vi "Main-PSD+EQP_YCC.vi"() -> ()   [LabVIEW 2014]
uses:
  Main-Stage-PI/(Global) Current handle and LaserPower_YCC.vi
  <vilib>/DAQmx/create/channels.llb/DAQmx Create Channel (AI-Voltage-Basic).vi
  <vilib>/DAQmx/configure/timing.llb/DAQmx Timing (Sample Clock).vi
  <vilib>/DAQmx/read.llb/DAQmx Read (Analog 2D DBL NChan NSamp).vi
panel:
  in  "Notch Filter On?":bool
  out "QPD raw(V) xyz":dbl[][](array[numeric])
  out "kx (pN/nm)":dbl
  in  "Who's Data":enum16{"YCC", "PYW", "LCH", "YYH"}(ring)
  in  "Save?":bool
  out "Frequency (Hz)\n0,df, 2df,...(n/2-1)Fs":dbl[](array[numeric])
  in  "Temperature (C)":dbl=22.0
  out "df (freq. resolution) Hz":dbl
  in  "record time per cycle (s)":dbl=0.125
  in  "EQP on?":bool
  out "Beta (V/um)":dbl[](array[numeric])
  out "Varicance (V^2)":dbl[](array[numeric])
  out "y-variance (V)":dbl format="%0.2f"
  out "x-variance (V)":dbl format="%0.2f"
  out "Y-conversion factor (V/um)":dbl
  out "X-conversion factor (V/um)":dbl
  out "EQP-Trap Stiffness (pN/nm)":dbl[](array[numeric])
  out "best fit parameters-y":dbl[](array[numeric])
  out "best fit parameters-z":dbl[](array[numeric])
  out "best fit parameters-x":dbl[](array[numeric])
  in  "Fit z?":bool
  in  "Fit y?":bool
  out "best nonlinear fit PSDz":dbl[](array[numeric])
  out "best nonlinear fit PSDy":dbl[](array[numeric])
  out "best nonlinear fit PSDx":dbl[](array[numeric])
  in  "Custum Fs (Hz)":i32
  in  "Focal shift factor":dbl=1.22
  out "best fit parameters":dbl[][](array[numeric])
  out "kx/kz":dbl
  in  "Freq End Cut":dbl=60000.0
  in  "Freq Strat Cut":dbl=10.0
  out "Trap Stiffness (pN/nm)":dbl[](array[numeric])
  in  "bead height (um)":dbl=2.0
  in  "bead radius (um)":dbl=0.515
  out "PSDz":dbl[](array[numeric])
  out "PSDy":dbl[](array[numeric])
  out "PSDx":dbl[](array[numeric])
  out "Frequency (Hz)\n0,df, 2df,...1/2Fs":dbl[](array[numeric])
  in  "Tab Control":enum32{"PSD x & y", "PSD x & z"}(tab)
  out "PSD x & y":T1(graph)
  out "PSD x & z":T2(graph)
  out "Corner Frequency (Hz)\n(fx,fy,fz)":dbl[](array[numeric])
  in  "Fit Lorentz PSD?":bool=TRUE
  out "Avg. PSD":dbl[][](array[numeric])
  out "# of PSD sum":i32
  in  "# of PSD Avg.":dbl=50.0
  in  "stop to fit":bool
  in  "T=NI made PSD\nF=YCC made PSD":bool
  out "Sampling rate (Hz)":i32
  in  "physical channels":tag="Dev2/ai2, Dev2/ai0, Dev2/ai16"
  in  "Sampling Rate (Hz)":T3(ring)=enum."131072"
  # "Fc=80k for fs=131072Hz"
  # "x"
  # "y"
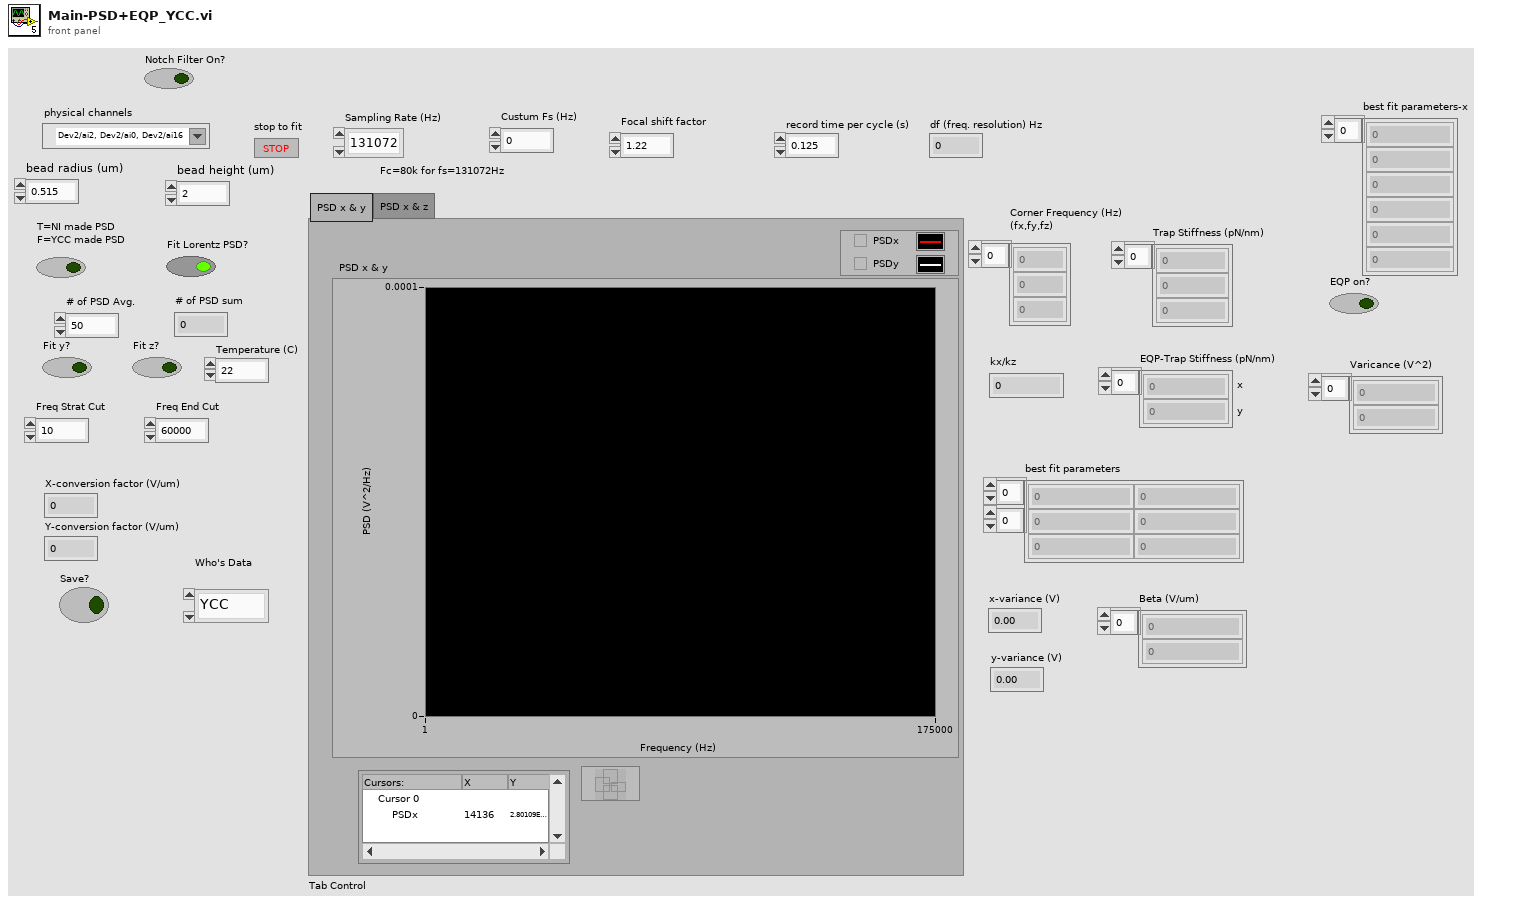
[diagram p1: front panel]
types:
  T1 = cluster{"Frequency (Hz)\ndf, 2df,...1/2Fs":dbl[], "PSDy":dbl[]}[]
  T2 = cluster{"Frequency (Hz)\ndf, 2df,...1/2Fs":dbl[], "PSDz":dbl[]}[]
  T3 = enum16{"custum", "16384", "32768", "65536", "131072", "262144"}
  T4 = cluster{"Frequency (Hz)\n0,df, 2df,...1/2Fs":dbl[], "PSDx":dbl[]}
  T5 = cluster{"Frequency (Hz)\n0,df, 2df,...1/2Fs":dbl[], "PSDz":dbl[]}
  T6 = cluster{"Frequency (Hz)\n0,df, 2df,...1/2Fs":dbl[], "PSDy":dbl[]}
  T7 = cluster{"Frequency (Hz)\n0,df, 2df,...1/2Fs":dbl[], "PSDz":dbl[]}[]
  T8 = cluster{"Frequency (Hz)\n0,df, 2df,...1/2Fs":dbl[], "PSDy":dbl[]}[]
  T9 = cluster{"Frequency (Hz)\n0,df, 2df,...1/2Fs":dbl[], "best nonlinear fit PSDz":dbl[]}
  T10 = cluster{"Frequency (Hz)\n0,df, 2df,...1/2Fs":dbl[], "best nonlinear fit PSDx":dbl[]}
  T11 = cluster{"Frequency (Hz)\n0,df, 2df,...1/2Fs":dbl[], "best nonlinear fit PSDy":dbl[]}
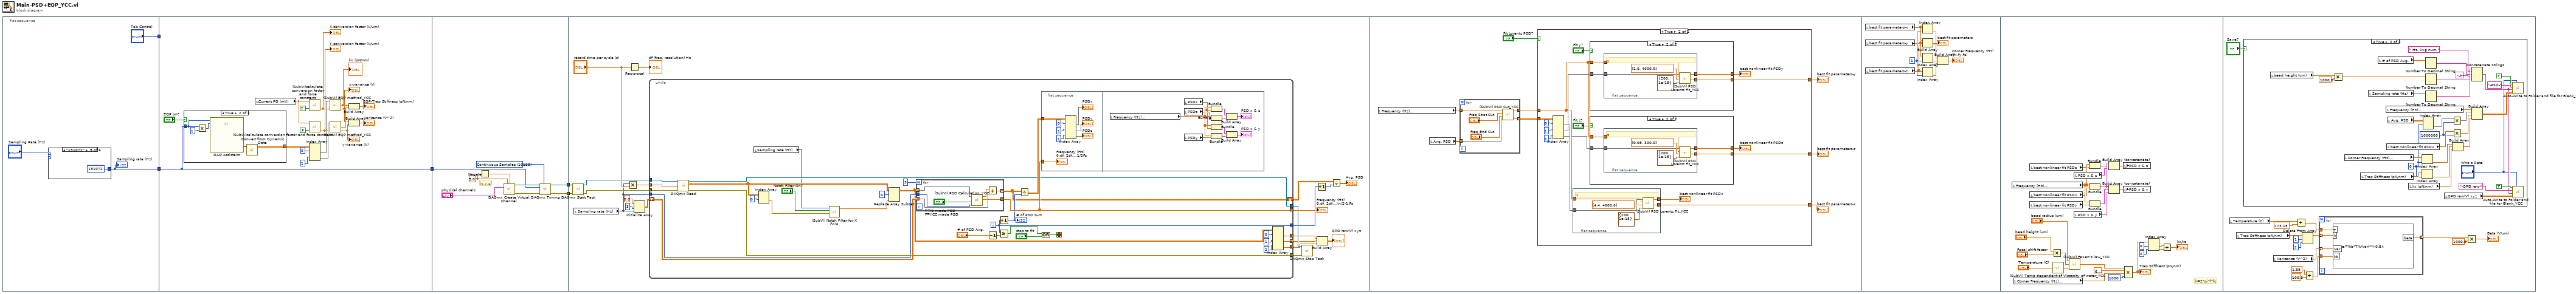
[diagram p0: block diagram]
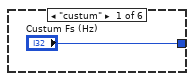
[diagram p2: hidden frame]
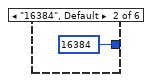
[diagram p3: hidden frame]
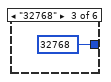
[diagram p4: hidden frame]
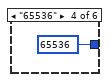
[diagram p5: hidden frame]
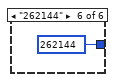
[diagram p6: hidden frame]
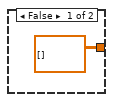
[diagram p7: hidden frame]
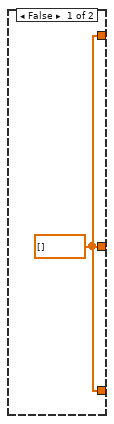
[diagram p8: hidden frame]
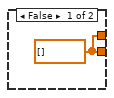
[diagram p9: hidden frame]
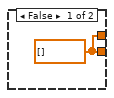
[diagram p10: hidden frame]
diagram:
  n1 = flat-sequence {
    tunnel: [w7] -> w3
    tunnel: ["Tab Control"] -> w1
    tunnel: w3 -> [w32]
    tunnel: [w32] -> w2
    tunnel: w1 -> [_]
    tunnel: w2 -> [w45]
    tunnel: [w42] -> w5
    tunnel: [w41] -> w4
    tunnel: w5 -> [w69]
    tunnel: w4 -> [w68]
    frame #0 {
      n2 = case shown="\"131072\"" "Sampling Rate (Hz)" {
        tunnel: ["Custum Fs (Hz)" 16384 32768 65536 131072 262144] -> w7
        frame "custum" {
        }
        frame "16384", Default {
        }
        frame "32768" {
        }
        frame "65536" {
        }
        frame "131072" {
        }
        frame "262144" {
        }
      }
      "Sampling rate (Hz)" <- w7
    }
    frame #1 {
      n3 = case shown="True" "EQP on?" {
        tunnel: w32 -> [_ w38]
        tunnel: [dbl[][] [] ("Array") w34] -> w21
        frame False {
        }
        frame True {
          n4 = Multiply(x=w38, y=1) -> (x*y=w36:i32)
          n5 = call "DAQ Assistant"("rate"=w38, "number of samples"=w36) -> ("data"=w35:dynamicdata)  [unwired: 15 in, 2 out]
          n6 = call "Convert from Dynamic Data"("Dynamic Data Type"=w35) -> ("Array"=w34:dbl[][])  [unwired: 3 in]
        }
      }
      n7 = global read "(Global) Current handle and LaserPower_YCC.vi" "Current PD (mV)"() -> (w18:dbl)
      n8 = Index Array(array=w21, index (row) #1=0 ("index (row)"), index (row) #2=1 ("index (row)")) -> (element #1=w29:dbl[], element #2=w28:dbl[])  [unwired: 2 in]
      n9 = call "(SubVI)calculate conversion factor and force constant.vi"("X=T\nY=F"=TRUE ("X=T\nY=F"), "laser power (mW)"=w18) -> ("conversion factor (V/um)"=w17:dbl)  [unwired: 2 in, 1 out]
      "X-conversion factor (V/um)" <- w17
      n10 = call "(SubVI)calculate conversion factor and force constant.vi"("X=T\nY=F"=FALSE ("X=T\nY=F"), "laser power (mW)"=w18) -> ("conversion factor (V/um)"=w19:dbl)  [unwired: 2 in, 1 out]
      "Y-conversion factor (V/um)" <- w19
      n11 = call "(SubVI) EQP method_YCC.vi"("Sensitivity (V/um)"=w17, "position (V)"=w29) -> ("variance (V)"=w24:dbl, "k (pN/nm)"=w27:dbl)  [unwired: 2 in]
      "x-variance (V)" <- w24
      "kx (pN/nm)" <- w27
      n12 = call "(SubVI) EQP method_YCC.vi"("Sensitivity (V/um)"=w19, "position (V)"=w28) -> ("variance (V)"=w23:dbl, "k (pN/nm)"=w26:dbl)  [unwired: 2 in]
      "y-variance (V)" <- w23
      n13 = Build Array(w27, w26) -> (→"EQP-Trap Stiffness (pN/nm)":dbl[])
      n14 = Build Array(w24, w23) -> (→"Varicance (V^2)":dbl[])
    }
    frame #2 {
      w40 = 5.0 ("maximum value")
      w43 = 10123 items=["Finite Samples"=10178, "Continuous Samples"=10123, "Hardware Timed Single Point"=12522] ("sample mode")
      # "(x,y,z)"
      n15 = Negate(x=w40) -> (-x=w39:dbl)
      n16 = call-poly <vilib>:"DAQmx Create Virtual Channel.vi"("maximum value"=w40, "minimum value"=w39, "physical channels"="physical channels") -> ("task out"=w46:refnum<k21>, "error out"=w44:errorcluster)  [unwired: 11 in]
      n17 = call-poly <vilib>:"DAQmx Timing.vi"("task/channels in"=w46, "sample mode"=w43, "rate"=w45, "error in"=w44) -> ("task out"=w42:refnum<k21>, "error out"=w41:errorcluster)  [unwired: 10 in]
    }
    frame #3 {
      n18 = call <vilib>:"DAQmx Start Task.vi"("task/channels in"=w69, "error in"=w68) -> ("task out"=w67:refnum<k21>, "error out"=w66:errorcluster)  [unwired: 12 in]
      n19 = local read "Sampling rate (Hz)"() -> (w52:i32)
      n20 = Multiply(x=w52, y="record time per cycle (s)") -> (x*y=w55:dbl)
      n21 = Reciprocal(x="record time per cycle (s)") -> (1/x=→"df (freq. resolution) Hz":dbl)
      n22 = Initialize Array(0.0 ("element"), 3 ("dimension size"), w52) -> (w63:dbl[][])
      n23 = while {
        tunnel: w67 -> [w101]
        tunnel: w66 -> [w100]
        shift-right: [w86] -> w56
        shift-left: w63 -> [w99]
        tunnel: [w90] -> w59
        tunnel: w55 -> [w85]
        tunnel: [w91] -> w62
        tunnel: [w89] -> w58
        tunnel: [w88] -> w57
        tunnel: w52 -> [w84]
        tunnel: [w80] -> w51 mode=concatenating
        tunnel: [w79] -> w50 mode=concatenating
        tunnel: [w78] -> w49 mode=concatenating
        i -> [w91]
        stop <- w94 stop-if-true
        n24 = call-poly <vilib>:"DAQmx Read.vi"("task/channels in"=w101, "number of samples per channel"=w85, "error in"=w100) -> ("task out"=w89:refnum<k21>, "data"=w75:dbl[][], "error out"=w88:errorcluster)  [unwired: 10 in]
        n25 = local read "Sampling rate (Hz)"() -> (w72:i32)
        n26 = Index Array(array=w75, index (row)=0) -> (element=w70:dbl[])  [unwired: 1 in]
        n27 = call "(SubVI) Notch Filter for X Axis.vi"("Sampling rate (Hz)"=w72, "Notch Filter On?"="Notch Filter On?", "data"=w70) -> ("Filtered Data"=w73:dbl[])  [unwired: 5 in]
        n28 = Replace Array Subset(array=w75, new element=w73, index (row)=0) -> (w74:dbl[][])  [unwired: 1 in]
        n29 = for {
          N: 3 -> [_]
          tunnel: w74 -> [w126] mode=indexing
          tunnel: w84 -> [w120]
          tunnel: [w123] -> w90
          tunnel: [w122] -> w86 mode=indexing
          tunnel: w99 -> [w121] mode=indexing
          n30 = call "(SubVI) PSD Calculation_YCC.vi"("sampling frequency (Hz)"=w120, "T=NI made PSD\nF=YCC made PSD"="T=NI made PSD\nF=YCC made PSD", "QPD data"=w126) -> ("Frequency (Hz)\n0,df, 2df,...(n/2-1)Fs"=w123:dbl[], "Power Spectrum (V^2 rms) (V^2/Hz)"=w124:dbl[])  [unwired: 3 in]
          n31 = Add(x=w124, y=w121) -> (x+y=w122:dbl[])
        }
        n32 = Decrement(x="# of PSD Avg.") -> (x-1=w96:dbl)
        n33 = Increment(x=w91) -> (x+1=w87:i32)
        "# of PSD sum" <- w87
        n34 = Greater Or Equal?(x=w91, y=w96) -> (x >= y?=w95:bool)
        n35 = Divide(x=w86, y=w87) -> (x/y=w92:dbl[][])
        n36 = Or(x=w95, y="stop to fit") -> (x .or. y?=w94:bool)
        n37 = flat-sequence {
          tunnel: w92 -> [w106]
          tunnel: w90 -> [w103]
          frame #0 {
            n38 = Index Array(array=w106, index (row) #1=0 ("index (row)"), index (row) #2=1 ("index (row)"), index (row) #3=2 ("index (row)")) -> (element #1=→"PSDx":dbl[], element #2=→"PSDy":dbl[], element #3=→"PSDz":dbl[])  [unwired: 3 in]
            "Frequency (Hz)\n0,df, 2df,...1/2Fs" <- w103
          }
          frame #1 {
            n39 = local read "Frequency (Hz)\n0,df, 2df,...1/2Fs"() -> (w115:dbl[])
            n40 = local read "PSDx"() -> (w110:dbl[])
            n41 = local read "PSDz"() -> (w111:dbl[])
            n42 = local read "PSDy"() -> (w116:dbl[])
            n43 = Bundle("Frequency (Hz)\n0,df, 2df,...1/2Fs"=w115, "PSDx"=w110) -> (w113:T4)  [unwired: 1 in]
            n44 = Bundle("Frequency (Hz)\n0,df, 2df,...1/2Fs"=w115, "PSDz"=w111) -> (w112:T5)  [unwired: 1 in]
            n45 = Bundle("Frequency (Hz)\n0,df, 2df,...1/2Fs"=w115, "PSDx"=w110) -> (w117:T4)  [unwired: 1 in]
            n46 = Bundle("Frequency (Hz)\n0,df, 2df,...1/2Fs"=w115, "PSDy"=w116) -> (w118:T6)  [unwired: 1 in]
            n47 = Build Array(w113, w112) -> (→"PSD x & z":T7)
            n48 = Build Array(w117, w118) -> (→"PSD x & y":T8)
          }
        }
        n49 = Index Array(array=w74, index (row) #1=0 ("index (row)"), index (row) #2=1 ("index (row)"), index (row) #3=2 ("index (row)")) -> (element #1=w80:dbl[], element #2=w79:dbl[], element #3=w78:dbl[])  [unwired: 3 in]
      }
      "Frequency (Hz)\n0,df, 2df,...(n/2-1)Fs" <- w59
      n50 = call <vilib>:"DAQmx Stop Task.vi"("task/channels in"=w58, "error in"=w57) -> ()  [unwired: 12 in, 2 out]
      n51 = Increment(x=w62) -> (x+1=w61:i32)
      n52 = Build Array(w51, w50, w49) -> (→"QPD raw(V) xyz":dbl[][])
      n53 = Divide(x=w56, y=w61) -> (x/y=→"Avg. PSD":dbl[][])
    }
    frame #4 {
      n54 = local read "Frequency (Hz)\n0,df, 2df,...(n/2-1)Fs"() -> (w128:dbl[])
      n55 = local read "Avg. PSD"() -> (w127:dbl[][])
      n56 = for {
        tunnel: w127 -> [w140] mode=indexing
        tunnel: w128 -> [w139]
        tunnel: [w138] -> w133
        tunnel: [w137] -> w132 mode=indexing
        n57 = call "(SubVI) PSD Cut_YCC.vi"("PSD"=w140, "Freq End Cut"="Freq End Cut", "Freq Strat Cut"="Freq Strat Cut", "Frequency (Hz)"=w139) -> ("PSD Cut"=w137:dbl[], "Freq Cut"=w138:dbl[])  [unwired: 2 in]
      }
      n58 = case shown="True" "Fit Lorentz PSD?" {
        tunnel: w132 -> [_ w157]
        tunnel: w133 -> [_ w150]
        tunnel: [w141 w145] -> w131
        tunnel: [w141 w144] -> w130
        tunnel: [w141 w143] -> w129
        frame False {
          w141 = dbl[] []
        }
        frame True {
          n59 = Index Array(array=w157, index (row) #1=0 ("index (row)"), index (row) #2=1 ("index (row)"), index (row) #3=2 ("index (row)")) -> (element #1=w153:dbl[], element #2=w152:dbl[], element #3=w151:dbl[])  [unwired: 3 in]
          n60 = flat-sequence {
            tunnel: w153 -> [w183]
            tunnel: w150 -> [w182]
            tunnel: [w181] -> w143
            tunnel: [w180] -> w142
            frame #0 {
              # "x"
              n61 = call "(SubVI) PSD Lorentz Fit_YCC.vi"("termination"=cluster{"max iteration":i32, "tolerance":dbl} {"max iteration"=200, "tolerance"=1e-15}, "initial parameters"=dbl[] [4.4, 4000.0], "Frequency (Hz)"=w182, "PSD (Vrms^2)"=w183) -> ("best fit parameters"=w181:dbl[], "best nonlinear fit PSD"=w180:dbl[])  [unwired: 2 in]
            }
          }
          n62 = case shown="True" "Fit y?" {
            tunnel: w152 -> [_ w173]
            tunnel: w150 -> [_ w172]
            tunnel: [w169 w171] -> w145
            tunnel: [w169 w170] -> w149
            frame False {
              w169 = dbl[] [] ("best nonlinear fit PSD")
            }
            frame True {
              n63 = flat-sequence {
                tunnel: w173 -> [w177]
                tunnel: w172 -> [w176]
                tunnel: [w175] -> w171
                tunnel: [w174] -> w170
                frame #0 {
                  # "y"
                  n64 = call "(SubVI) PSD Lorentz Fit_YCC.vi"("termination"=cluster{"max iteration":i32, "tolerance":dbl} {"max iteration"=200, "tolerance"=1e-15}, "initial parameters"=dbl[] [1.0, 4000.0], "Frequency (Hz)"=w176, "PSD (Vrms^2)"=w177) -> ("best fit parameters"=w175:dbl[], "best nonlinear fit PSD"=w174:dbl[])  [unwired: 2 in]
                }
              }
            }
          }
          "best nonlinear fit PSDy" <- w149
          n65 = case shown="True" "Fit z?" {
            tunnel: w151 -> [_ w162]
            tunnel: w150 -> [_ w161]
            tunnel: [w158 w160] -> w144
            tunnel: [w158 w159] -> w148
            frame False {
              w158 = dbl[] [] ("best nonlinear fit PSD")
            }
            frame True {
              n66 = flat-sequence {
                tunnel: w162 -> [w166]
                tunnel: w161 -> [w165]
                tunnel: [w164] -> w160
                tunnel: [w163] -> w159
                frame #0 {
                  # "z"
                  n67 = call "(SubVI) PSD Lorentz Fit_YCC.vi"("termination"=cluster{"max iteration":i32, "tolerance":dbl} {"max iteration"=200, "tolerance"=1e-15}, "initial parameters"=dbl[] [0.05, 300.0], "Frequency (Hz)"=w165, "PSD (Vrms^2)"=w166) -> ("best fit parameters"=w164:dbl[], "best nonlinear fit PSD"=w163:dbl[])  [unwired: 2 in]
                }
              }
            }
          }
          "best nonlinear fit PSDz" <- w148
          "best nonlinear fit PSDx" <- w142
        }
      }
      "best fit parameters-y" <- w131
      "best fit parameters-z" <- w130
      "best fit parameters-x" <- w129
    }
    frame #5 {
      w192 = 1 ("index")
      n68 = local read "best fit parameters-x"() -> (w193:dbl[])
      n69 = local read "best fit parameters-y"() -> (w191:dbl[])
      n70 = local read "best fit parameters-z"() -> (w190:dbl[])
      n71 = Index Array(array=w193, index=w192) -> (element=w189:dbl)
      n72 = Build Array(w193, w191, w190) -> (→"best fit parameters":dbl[][])
      n73 = Index Array(array=w191, index=w192) -> (element=w188:dbl)
      n74 = Index Array(array=w190, index=w192) -> (element=w187:dbl)
      n75 = Build Array(w189, w188, w187) -> (→"Corner Frequency (Hz)\n(fx,fy,fz)":dbl[])
    }
    frame #6 {
      # "k=2*pi*f*fc"
      n76 = local read "Frequency (Hz)\n0,df, 2df,...1/2Fs"() -> (w217:dbl[])
      n77 = local read "Corner Frequency (Hz)\n(fx,fy,fz)"() -> (w195:dbl[])
      n78 = local read "best nonlinear fit PSDz"() -> (w198:dbl[])
      n79 = local read "best nonlinear fit PSDx"() -> (w200:dbl[])
      n80 = local read "best nonlinear fit PSDy"() -> (w199:dbl[])
      n81 = Multiply(x="bead height (um)", y="Focal shift factor") -> (x*y=w201:dbl)
      n82 = call "(SubVI) Temp dependent of Viscosity of water_YCC.vi"("Temperature (C)"="Temperature (C)") -> ("Viscosity (mPa*s)"=w196:dbl)  [unwired: 4 in]
      n83 = call "(SubVI) Faxen's law_YCC.vi"("viscosity (cP)"=w196, "bead height (um)"=w201, "bead radius (um)"="bead radius (um)") -> ("Faxen's law of friction coefficient (N/(m/s))"=w219:dbl)  [unwired: 2 in]
      n84 = local read "PSD x & z"() -> (w211:T2)
      n85 = local read "PSD x & y"() -> (w210:T1)
      n86 = Bundle("Frequency (Hz)\n0,df, 2df,...1/2Fs"=w217, "best nonlinear fit PSDz"=w198) -> (w213:T9)  [unwired: 1 in]
      n87 = Bundle("Frequency (Hz)\n0,df, 2df,...1/2Fs"=w217, "best nonlinear fit PSDx"=w200) -> (w214:T10)  [unwired: 1 in]
      n88 = Bundle("Frequency (Hz)\n0,df, 2df,...1/2Fs"=w217, "best nonlinear fit PSDy"=w199) -> (w216:T11)  [unwired: 1 in]
      n89 = Build Array (concatenate)(w214, w213, w211) -> (w212:T2)
      n90 = Build Array (concatenate)(w214, w216, w210) -> (w215:T1)
      n91 = local write "PSD x & z"(w212) -> ()
      n92 = local write "PSD x & y"(w215) -> ()
      n93 = Compound Arithmetic op=MULTIPLY(w219, 6.283185307179586, w195, 1000 ("Numeric")) -> (w209:dbl[])
      "Trap Stiffness (pN/nm)" <- w209
      n94 = Index Array(array=w209, index #1=0 ("index"), index #2=2 ("index")) -> (element #1=w206:dbl, element #2=w205:dbl)
      n95 = Divide(x=w206, y=w205) -> (x/y=→"kx/kz":dbl)
    }
    frame #7 {
      n96 = local read "Temperature (C)"() -> (w223:dbl)
      n97 = local read "Trap Stiffness (pN/nm)"() -> (w231:dbl[])
      n98 = case shown="True" "Save?" {
        frame False {
        }
        frame True {
          w257 = 1000000 ("Numeric")
          w264 = 0 ("index (row)")
          n99 = local read "bead height (um)"() -> (w246:dbl)
          n100 = Multiply(x=w246, y=1000.0) -> (x*y=w244:dbl)
          n101 = local read "Corner Frequency (Hz)\n(fx,fy,fz)"() -> (w265:dbl[])
          n102 = local read "Trap Stiffness (pN/nm)"() -> (w266:dbl[])
          n103 = local read "Sampling rate (Hz)"() -> (w252:i32)
          n104 = local read "# of PSD Avg."() -> (w249:dbl)
          n105 = local read "Frequency (Hz)\n0,df, 2df,...(n/2-1)Fs"() -> (w268:dbl[])
          n106 = local read "best nonlinear fit PSDx"() -> (w260:dbl[])
          n107 = local read "Avg. PSD"() -> (w267:dbl[][])
          n108 = local read "kx (pN/nm)"() -> (w247:dbl)
          n109 = Index Array(array=w265, index=w264) -> (element=w263:dbl)
          n110 = Index Array(array=w266, index=w264) -> (element=w262:dbl)
          n111 = Index Array(array=w267, index (row)=w264) -> (element=w258:dbl[])  [unwired: 1 in]
          n112 = Number To Decimal String(number=w249) -> (decimal integer string=w248:string)  [unwired: 1 in]
          n113 = Number To Decimal String(number=w244) -> (decimal integer string=w243:string)  [unwired: 1 in]
          n114 = Number To Decimal String(number=w252) -> (decimal integer string=w251:string)  [unwired: 1 in]
          n115 = local read "QPD raw(V) xyz"() -> (w238:dbl[][])
          n116 = Multiply(x=w258, y=w257) -> (x*y=w256:dbl[])
          n117 = Multiply(x=w260, y=w257) -> (x*y=w259:dbl[])
          n118 = Build Array(w263, w262, w247) -> (w261:dbl[])
          n119 = Concatenate Strings(w251, " Hz- Avg num " ("string"), w248, "-h" ("string"), w243) -> (w239:string)
          n120 = Build Array(w268, w256, w259, w261) -> (w255:dbl[][])
          n121 = call "Auto-Write to Folder and file for Blank_YCC.vi"("Who's Data"="Who's Data", "data to be saved"=w255, "File name add to the end \n(height)"=w239, "Title"="-PSD-", "Save?"=TRUE) -> ()  [unwired: 3 in, 2 out]
          n122 = call "Auto-Write to Folder and file for Blank_YCC.vi"("Who's Data"="Who's Data", "data to be saved"=w238, "File name add to the end \n(height)"=w239, "Title"="-QPD raw-", "Save?"=TRUE) -> ()  [unwired: 3 in, 2 out]
        }
      }
      n123 = local read "Varicance (V^2)"() -> (w227:dbl[])
      n124 = Add(x=w223, y=273.15) -> (x+y=w233:dbl)
      n125 = Delete From Array(array=w231, length=1, index=2) -> (array with subset deleted=w228:dbl[])  [unwired: 1 out]
      n126 = Divide(x=1.38 ("input variable"), y=100.0) -> (x/y=w236:dbl)
      n127 = for {
        tunnel: w236 -> [w273]
        tunnel: w233 -> [w272]
        tunnel: w228 -> [w271] mode=indexing
        tunnel: w227 -> [w270] mode=indexing
        tunnel: [w269] -> w226 mode=indexing
        n128 = formula code="beta=(kb*T/k/Var)**(-0.5);"("T"=w272, "Var"=w270, "kb"=w273, "k"=w271) -> ("beta"=w269:dbl)
      }
      n129 = Multiply(x=w226, y=1000.0) -> (x*y=→"Beta (V/um)":dbl[])
    }
  }
